vi "validateScheduler.vi"(9 "Constraints":T1, 10 "Schedule":cluster{"time (s)":dbl, "setpoint ":dbl}[](array[cluster])) -> (1 "Invalid Input":bool, 2 "Valid Input":bool)   [LabVIEW 2018]
panel:
  out "Setpoint Array":dbl[](array[numeric])
  out "Frequency Array":dbl[](array[numeric])
  out "Time Array":dbl[](array[numeric])
  out "Max Rate":dbl
  out "Min Value":dbl
  out "Max Value":dbl
  # "For Debugging: Constraints and Variables"
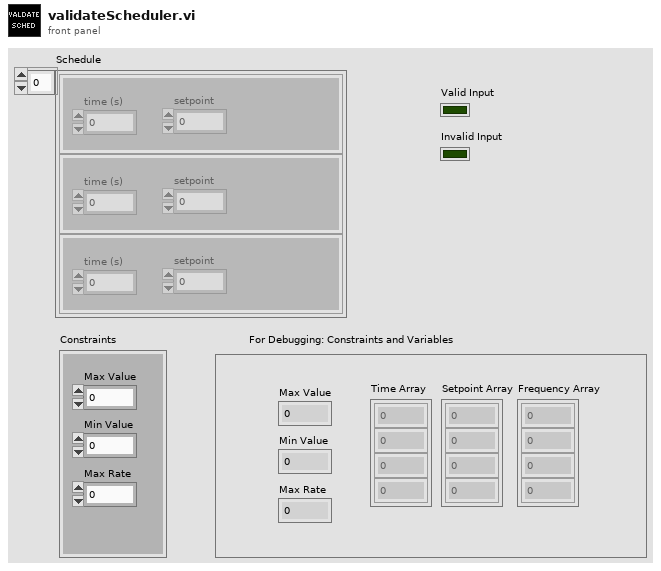
[diagram p1: front panel]
types:
  T1 = cluster{"Max Value":dbl, "Min Value":dbl, "Max Rate":dbl}
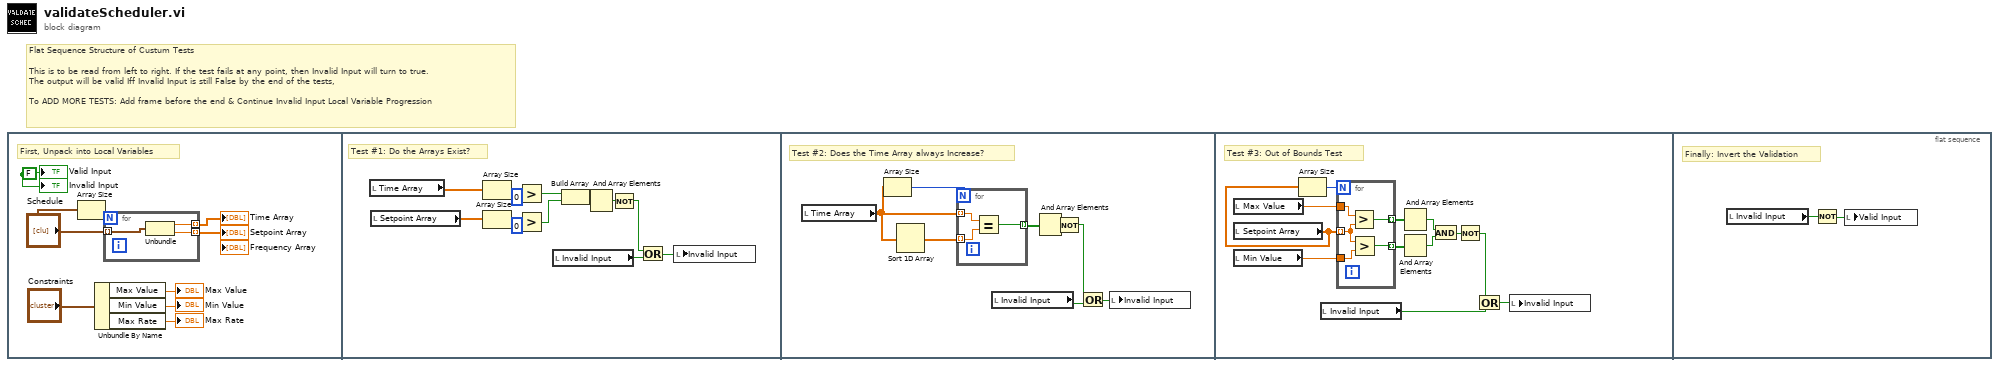
[diagram p0: block diagram]
diagram:
  # "Flat Sequence Structure of Custum Tests\n\nThis is to be read from left to right. If the test fails at any point, then Invalid Input will turn to true.\nThe output will be valid Iff Invalid Input is still False by the end of the tests,\n\nTo ADD MORE TESTS: Add frame before the end & Continue Invalid Input Local Variable Progression"
  n1 = flat-sequence {
    frame #0 {
      w9 = FALSE
      # "First, Unpack into Local Variables"
      n2 = Array Size(array="Schedule") -> (size(s)=w6:i32)
      n3 = Unbundle By Name("Constraints") -> ("Max Value"=→"Max Value":dbl, "Min Value"=→"Min Value":dbl, "Max Rate"=→"Max Rate":dbl)
      n4 = for {
        N: w6 -> [_]
        tunnel: "Schedule" -> [w12] mode=indexing
        tunnel: [w11] -> w8 mode=indexing
        tunnel: [w10] -> w1 mode=indexing
        n5 = Unbundle(w12) -> ("time (s)"=w11:dbl, "setpoint"=w10:dbl)
      }
      "Time Array" <- w8
      "Setpoint Array" <- w1
      "Valid Input" <- w9
      "Invalid Input" <- w9
    }
    frame #1 {
      # "Test #1: Do the Arrays Exist?"
      n6 = local read "Time Array"() -> (w25:dbl[])
      n7 = local read "Setpoint Array"() -> (w24:dbl[])
      n8 = Array Size(array=w25) -> (size(s)=w19:i32)
      n9 = Array Size(array=w24) -> (size(s)=w20:i32)
      n10 = Greater?(x=w19, y=0) -> (0:w18:bool)
      n11 = Greater?(x=w20, y=0) -> (0:w17:bool)
      n12 = local read "Invalid Input"() -> (w16:bool)
      n13 = Build Array(w18, w17) -> (w23:bool[])
      n14 = And Array Elements(Boolean array=w23) -> (logical AND=w13:bool)
      n15 = Not(x=w13) -> (.not. x?=w14:bool)
      n16 = Or(x=w14, y=w16) -> (x .or. y?=w15:bool)
      n17 = local write "Invalid Input"(w15) -> ()
    }
    frame #2 {
      # "Test #2: Does the Time Array always Increase?"
      n18 = local read "Time Array"() -> (w32:dbl[])
      n19 = Array Size(array=w32) -> (size(s)=w33:i32)
      n20 = Sort 1D Array(array=w32) -> (sorted array=w31:dbl[])
      n21 = for {
        N: w33 -> [_]
        tunnel: w32 -> [w36] mode=indexing
        tunnel: w31 -> [w35] mode=indexing
        tunnel: [w34] -> w30 mode=indexing
        n22 = Equal?(x=w36, y=w35) -> (x = y?=w34:bool)
      }
      n23 = local read "Invalid Input"() -> (w28:bool)
      n24 = And Array Elements(Boolean array=w30) -> (logical AND=w27:bool)
      n25 = Not(x=w27) -> (.not. x?=w26:bool)
      n26 = Or(x=w26, y=w28) -> (x .or. y?=w29:bool)
      n27 = local write "Invalid Input"(w29) -> ()
    }
    frame #3 {
      # "Test #3: Out of Bounds Test"
      n28 = local read "Max Value"() -> (w46:dbl)
      n29 = local read "Setpoint Array"() -> (w45:dbl[])
      n30 = local read "Min Value"() -> (w47:dbl)
      n31 = Array Size(array=w45) -> (size(s)=w48:i32)
      n32 = local read "Invalid Input"() -> (w39:bool)
      n33 = for {
        N: w48 -> [_]
        tunnel: w47 -> [w51]
        tunnel: w46 -> [w53]
        tunnel: w45 -> [w52] mode=indexing
        tunnel: [w50] -> w44 mode=indexing
        tunnel: [w49] -> w43 mode=indexing
        n34 = Greater?(x=w53, y=w52) -> (0:w50:bool)
        n35 = Greater?(x=w52, y=w51) -> (0:w49:bool)
      }
      n36 = And Array Elements(Boolean array=w44) -> (logical AND=w41:bool)
      n37 = And Array Elements(Boolean array=w43) -> (logical AND=w42:bool)
      n38 = And(x=w41, y=w42) -> (x .and. y?=w38:bool)
      n39 = Not(x=w38) -> (.not. x?=w37:bool)
      n40 = Or(x=w37, y=w39) -> (x .or. y?=w40:bool)
      n41 = local write "Invalid Input"(w40) -> ()
    }
    frame #4 {
      # "Finally: Invert the Validation"
      n42 = local read "Invalid Input"() -> (w55:bool)
      n43 = Not(x=w55) -> (.not. x?=w54:bool)
      n44 = local write "Valid Input"(w54) -> ()
    }
  }
